vi "List Azure Queues.vi"() -> ()   [LabVIEW 2015]
doc: "Demonstrates how to list all Amazon SQS queues created by an authenticated user."
uses:
  Core/Azure Credentials.ctl
  Core/NI_Azure_Core.lvlib
  Core/Session/Session.lvclass
  Queue/NI_Azure_Queue.lvlib
panel:
  in  "Access Key":string
  in  "Storage Account Name":string
  out "Queues":i32(listbox)
  # "Overview: Demonstrates how to list all Azure queues associated with a storage account.\nRequirements: NI Cloud Toolkit for Azure and a registered Microsoft Azure account\nInstructions:\n1. Specify the Storage Account Name and Access Key for your Azure account. You can create an account at http://azure.microsoft.com.\n2. Run the VI. All the queues associated with your account should be listed in the Queues indicator."
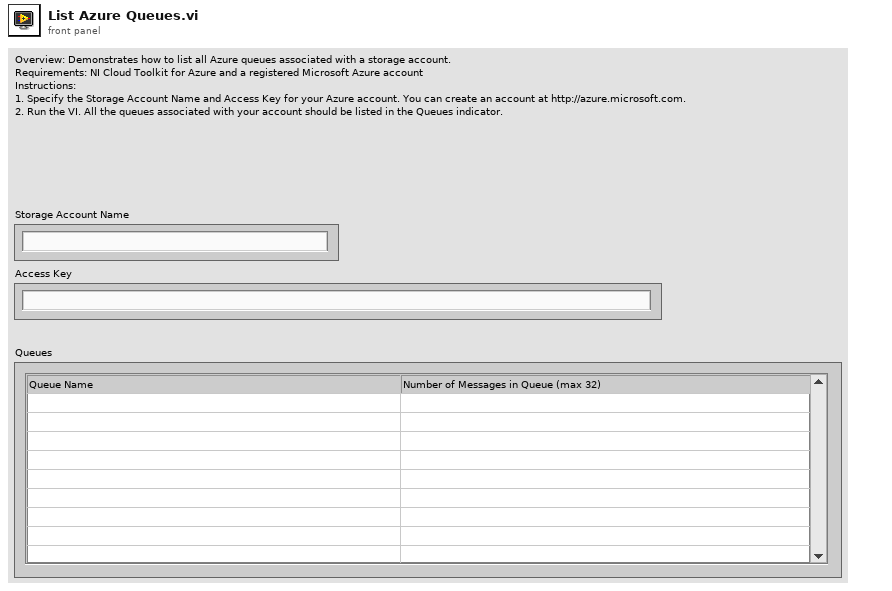
[diagram p1: front panel]
types:
  T1 = typedef "NI_Azure_Core.lvlib/Azure Credentials.ctl" = cluster{"Storage Account Name":string, "Access Key":string}
  T2 = typedef "NI_Azure_Queue.lvlib/Message.ctl" = cluster{"Message ID":string, "Insertion Time":string, "Expiration Time":string, "Pop Receipt":string, "Time Next Visible":string, "Dequeue Count":i32, "Message Text":string}
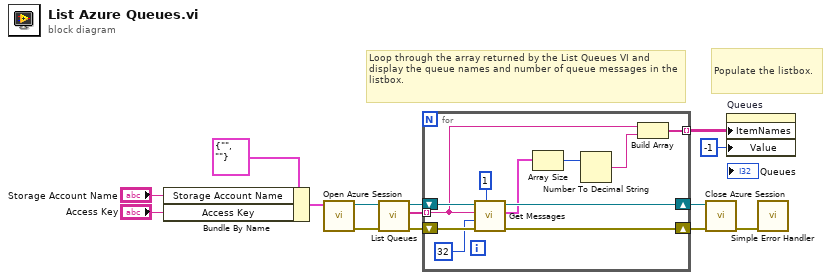
[diagram p0: block diagram]
diagram:
  # "Loop through the array returned by the List Queues VI and display the queue names and number of queue messages in the listbox."
  # "Populate the listbox."
  n1 = Bundle By Name(cluster=T1 {"Storage Account Name"="", "Access Key"=""} ("Credentials"), "Storage Account Name"="Storage Account Name", "Access Key"="Access Key") -> (w11:T1)
  n2 = call "Open Azure Session.vi"("Credentials"=w11) -> ("error out"=w10:errorcluster, "Azure Session"=w9:refnum<class "Session.lvclass">)  [unwired: 9 in]
  n3 = call "List Queues.vi"("error in (no error)"=w10, "Azure Session in"=w9) -> ("error out"=w7:errorcluster, "Queues"=w3:string[], "Azure Session out"=w8:refnum<class "Session.lvclass">)  [unwired: 7 in]
  n4 = for {
    shift-right: [w20] -> w6
    shift-left: w7 -> [w25]
    shift-right: [w21] -> w5
    shift-left: w8 -> [w24]
    tunnel: w3 -> [w18] mode=indexing
    tunnel: [w19] -> w1 mode=indexing
    n5 = call "Get Messages.vi"("Visibility timeout (30 seconds)"=u32 1, "error in (no error)"=w25, "Number of messages (1)"=u32 32, "Queue"=w18, "Azure Session in"=w24) -> ("error out"=w20:errorcluster, "Messages"=w17:T2[], "Azure Session out"=w21:refnum<class "Session.lvclass">)  [unwired: 4 in]
    n6 = Array Size(array=w17) -> (size(s)=w16:i32)
    n7 = Number To Decimal String(number=w16) -> (decimal integer string=w15:string)  [unwired: 1 in]
    n8 = Build Array(w18, w15) -> (w19:string[])
  }
  n9 = call "Close Azure Session.vi"("error in (no error)"=w6, "Azure Session"=w5) -> ("error out"=w4:errorcluster)  [unwired: 9 in]
  n10 = property on="Queues" class="MCListbox (strict)"("ItemNames"=w1, "Value"=-1 ("Queues")) -> ()  [unwired: 2 in, 2 out]
  n11 = call <vilib>:"Simple Error Handler.vi"("error in (no error)"=w4) -> ()  [unwired: 4 in, 5 out]
